vi "SelectUTChan.vi"(2 "错误输入（无错误）":errorcluster, 3 "指定的通道号":u8) -> (0 "错误输出":errorcluster)   [LabVIEW 2018]
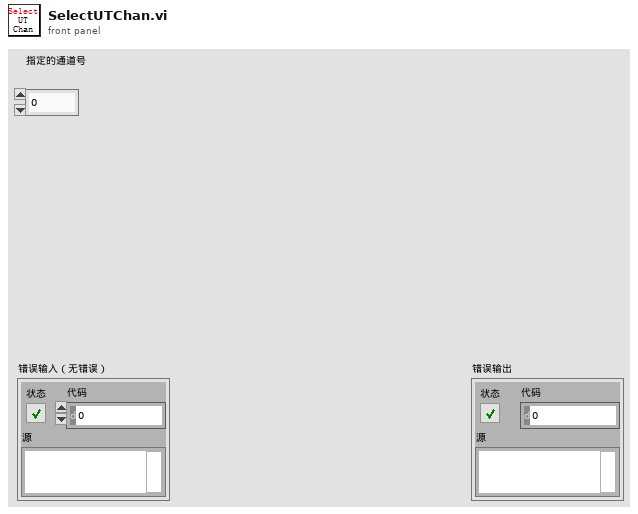
[diagram p1: front panel]
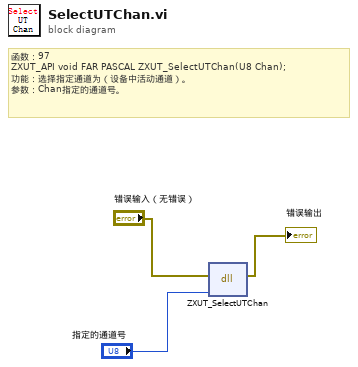
[diagram p0: block diagram]
diagram:
  # "函数：97\nZXUT_API void\tFAR PASCAL ZXUT_SelectUTChan(U8 Chan);\n功能：选择指定通道为（设备中活动通道）。\n参数：Chan指定的通道号。"
  n1 = dll-call lib="PTH2Rabs E软件项目超声超声子VI函数VI\tTCG处理ZXUTConfigMgr.dll" fn="ZXUT_SelectUTChan"(error in="错误输入（无错误）", "Chan"="指定的通道号") -> (error out=→"错误输出":errorcluster)  [unwired: 4 in, 1 out]
